vi "publishEventDetailedState.vi"(8 "error in (no error)":errorcluster, 11 "Model in":refnum<class "Model.lvclass">) -> (0 "error out":errorcluster, 3 "Model out":refnum<class "Model.lvclass">)   [LabVIEW 2016, in "Model.lvclass"]
uses:
  Model.lvclass
  Model.lvclass/Model.ctl
  Publisher/Publisher.lvclass/Publisher.ctl
  Communicator/M1M3SAL/M1M3SAL.lvclass/M1M3SAL.ctl
  Publisher/getM1M3SAL.vi
  Publisher/setM1M3SAL.vi
  Publisher/getEventDetailedState.vi
  Communicator/M1M3SAL/logDetailedState.vi
  Communicator/M1M3SAL/writeHeader.vi
  Communicator/M1M3SAL/writeDBL.vi
  Communicator/M1M3SAL/writeI32.vi
  Communicator/M1M3SAL/writeU8.vi
  Publisher/Publisher.lvclass
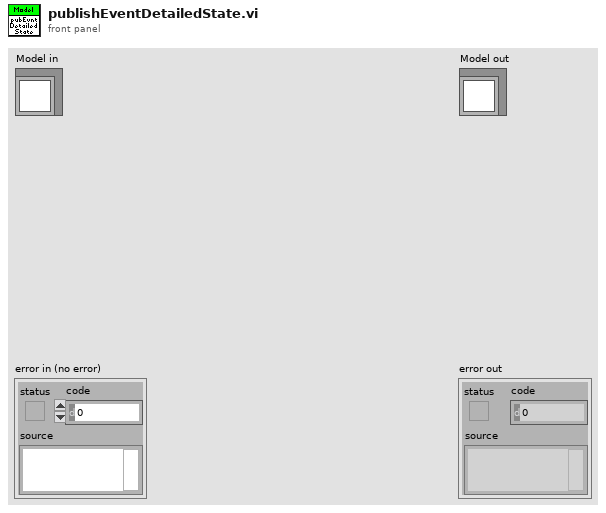
[diagram p1: front panel]
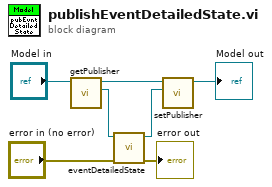
[diagram p0: block diagram]
diagram:
  n1 = call "getPublisher.vi"("Model in"="Model in") -> ("Publisher"=w2:refnum<class "Publisher.lvclass">, "Model out"=w6:refnum<class "Model.lvclass">)  [unwired: 9 in]
  n2 = call "eventDetailedState.vi"("error in (no error)"="error in (no error)", "Publisher in"=w2) -> ("error out"=→"error out":errorcluster, "Publisher out"=w1:refnum<class "Publisher.lvclass">)  [unwired: 8 in]
  n3 = call "setPublisher.vi"("Publisher"=w1, "Model in"=w6) -> ("Model out"=→"Model out":refnum<class "Model.lvclass">)  [unwired: 9 in]
